vi "Get Data from TCF.vi"(8 "error in (no error)":errorcluster, 10 "TCF Path":path, 11 "QFE3320 TCF Parser in":refnum<class "QPA TCF Parser.lvclass">) -> (0 "error out":errorcluster, 3 "QFE3320 TCF Parser out":refnum<class "QPA TCF Parser.lvclass">)   [LabVIEW 2016, in "QPA TCF Parser.lvlib" / "QPA TCF Parser.lvclass"]
uses:
  QPA TCF Parser.lvclass
  Controls/Worksheet Data.ctl
  QPA TCF Parser.lvclass/QPA TCF Parser.ctl
  <vilib>/addons/_office/excel.llb/Excel Get Data ([str]).vi
  <vilib>/Utility/NIReport.llb/NI_report.lvclass
  <vilib>/addons/_office/NI_ReportGenerationToolkit.lvlib
  <vilib>/Utility/NIReport.llb/Excel/NI_Excel.lvclass
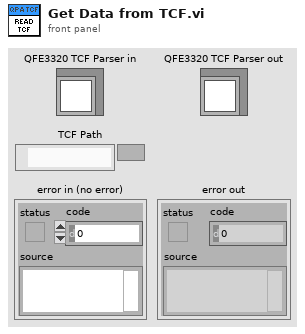
[diagram p1: front panel]
types:
  T1 = enum16{"Standard Report", "HTML", "Word", "Excel"}
  T2 = typedef "QPA TCF Parser.lvlib/QPA TCF Parser.lvclass/Worksheet Data.ctl" = cluster{"Worksheet Name":string, "Worksheet Data":string[][]}
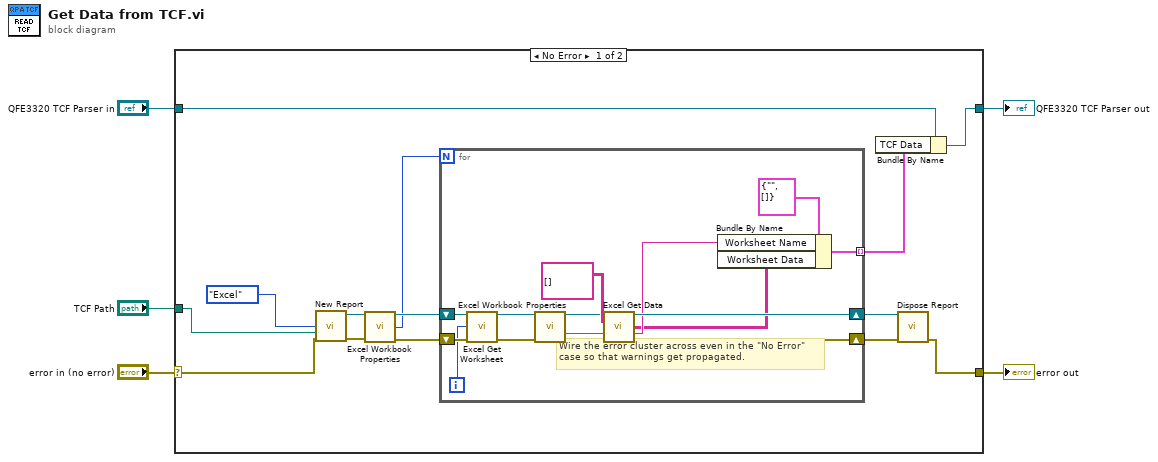
[diagram p0: block diagram]
diagram:
  n1 = case shown="No Error" "error in (no error)" {
    selector: "error in (no error)" -> [w11 w35]
    tunnel: [w10 w35] -> w4
    tunnel: [w7 w34] -> w2
    tunnel: "QFE3320 TCF Parser in" -> [w8 w34]
    tunnel: "TCF Path" -> [w6 _]
    frame No Error {
      # "Wire the error cluster across even in the \"No Error\"\ncase so that warnings get propagated."
      n2 = call <vilib>:"New Report.vi"("report type"=T1."Excel", "template (empty)"=w6, "error in (no error)"=w11) -> ("report out"=w18:refnum<class "NI_report.lvclass">, "error out"=w17:errorcluster)  [unwired: 11 in]
      n3 = call <vilib>:"Excel Workbook Properties.vi"("report in"=w18, "error in (no error)"=w17) -> ("report out"=w13:refnum<class "NI_report.lvclass">, "worksheets count"=w12:i32, "error out"=w16:errorcluster)  [unwired: 10 in, 1 out]
      n4 = for {
        N: w12 -> [_]
        shift-right: [w31] -> w14
        shift-left: w16 -> [w33]
        shift-right: [w32] -> w15
        shift-left: w13 -> [w29]
        tunnel: [w21] -> w9 mode=indexing
        i -> [w28]
        n5 = call <vilib>:"Excel Get Worksheet.vi"("report in"=w29, "worksheet index (0)"=w28, "error in (no error)"=w33) -> ("report out"=w25:refnum<class "NI_report.lvclass">, "error out"=w30:errorcluster)  [unwired: 11 in]
        n6 = call <vilib>:"Excel Workbook Properties.vi"("report in"=w25, "error in (no error)"=w30) -> ("report out"=w24:refnum<class "NI_report.lvclass">, "current worksheet name"=w23:string, "error out"=w26:errorcluster)  [unwired: 10 in, 1 out]
        n7 = call-poly <vilib>:"Excel Get Data.vi"("report in"=w24, "data type"=string[][] [], "error in (no error)"=w26) -> ("report out"=w32:refnum<class "NI_report.lvclass">, "data"=w22:string[][], "error out"=w31:errorcluster)  [unwired: 10 in]
        n8 = Bundle By Name(cluster=T2 {"Worksheet Name"="", "Worksheet Data"=[]} ("Worksheet Data"), "Worksheet Name"=w23, "Worksheet Data"=w22) -> (w21:T2)
      }
      n9 = Bundle By Name(cluster=w8, "TCF Data"=w9) -> (w7:refnum<class "QPA TCF Parser.lvclass">)
      n10 = call-dynamic "Dispose Report.vi"("report in"=w15, "error in (no error)"=w14) -> ("error out"=w10:errorcluster)  [unwired: 13 in]
    }
    frame Error {
    }
  }
  "error out" <- w4
  "QFE3320 TCF Parser out" <- w2
